vi "Test Functionality.vi"() -> ()   [LabVIEW 2014, in "Exponential Fit Library.lvlib" / "Fit Exponential.lvclass"]
doc: "This is a simle demonstration of the capabilities of the exponential fit class."
uses:
  Fit Exponential.lvclass
  Fit Exponential.lvclass/Fit Exponential.ctl
  Children/DFT1/DFT1.lvclass
  Children/DFT5/DFT5.lvclass
  Children/LRS/LRS.lvclass
  Read Output.vi
  <vilib>/Analysis/1siggen.llb/Ramp Pattern by Delta.vi
  <vilib>/Analysis/NI_AALBase.lvlib
panel:
  out "dt":u32
  out "Fit Output":T1={"e_tau"=99.90454010392875, "tau"=1.949455255190312, "B"=59.81343922735875, "A"=0.8596986263697382}
  in  "B":dbl=2.0
  in  "A":dbl=100.0
  in  "tau":dbl=60.0
  in  "Select Method":enum8{"DFT-1", "DFT-5", "LRS"}(ring)=enum."LRS"
  out "Error in Tau":dbl(graph)=0.8596986263697382
  out "Tau":dbl(graph)=59.81343922735875
  out "Exponential":dbl[](graph)=[105.19602012687483, 88.82122437603577, 94.96086320025637, 95.71453214801636, 95.59080261762062, 91.73977505742936, 85.3376433904598, 82.27233436951714, 84.01552271041503, 77.40281684842637, 81.73542102593571, 85.5916913851243, 79.70119362351942, 73.0659958752437, 78.56339184483366, 78.85934073769867, 67.70414981636233, 76.13121908133753, 69.24243068326123, 75.93686290556164, 63.65334373701221, 78.00875717550242, 70.49870699596495, 75.46168557646813, 72.57838577956375, 65.51622051875438, 65.06989722804512, 65.54430282784585, 55.741189323870316, 54.08478157966374, 54.58255994627164, 64.01000957310953, 50.199772855777525, 65.77049605242452, 54.32498195872571, 62.40495769659772, 60.547552705307, 60.78723411057597, 56.28221634523417, 57.45844769511123, 43.24267064639564, 54.33822050100301, 56.01714381694604, 42.26273032348696, 55.110548218852834, 39.62327233272855, 57.27265986474464, 39.45826734042453, 49.04520882302456, 54.61781894748323, 53.207409848009945, 42.66361091729411, 49.46109003839781, 48.91103509310124, 46.37787029719525, 48.57456698086692, 41.53558769893743, 34.09351700161767, 44.76087587046023, 34.82023460991957, 30.19579831795769, 38.392488493296355, 27.32886941188832, 38.96646638690362, 45.01641242989772, 38.82276973042363, 29.747464621972323, 35.70981436019103, 43.64893196471162, 24.812177457525692, 30.337410961802885, 34.34326852836734, 40.76943704863494, 36.247643405937595, 33.265050395620335, 32.44689219327494, 34.91970637396674, 33.625916966841515, 19.09799738264568, 18.557341036626255, 20.550492201879564, 27.987514461571667, 24.625099541142692, 29.030824648692366, 30.938021456477884, 32.36173983721376, 23.70605502436015, 31.50381194361505, 27.18395847183744, 19.109547699140037, 31.46399815246409, 32.4055920115639, 29.783303066363935, 21.176910913596856, 18.017561362062736, 29.097452111329016, 29.96401325470584, 12.471377487916932, 17.296472399075753, 19.037648942327067, 18.394059462335107, 10.519734089919409, 17.703505869750828, 15.300978961536357, 22.703770314965663, 19.39981126393128, 18.490932701971747, 26.69651222639837, 27.11347151333939, 21.851522164741706, 27.399987380327925, 26.153360943236436, 25.442547503709463, 18.612046341955406, 15.207507655743619, 17.246321867610533, 15.217487467609061, 16.415755701108175, 17.405877185115024, 9.643018876469466, 11.00197276324525, 17.78607754567581, 9.806038474233397, 13.89986279166466, 14.273651492614803, 23.97893894072294, 15.944196378192977, 19.462075911165755, 9.854457059328933, 11.511790216594417, 19.35752907658206, 12.241570925378142, 19.78650740157862, 15.923854316823356, 13.445190057683444, 11.305887529948066, 17.099190329363147, 12.408092598071667, 19.348867839911374, 19.68049621110516, 19.929585723285793, 9.176766049291864, 16.03337774975828, 10.72042467518554, 2.985353813851331, 8.80880342347193, 20.43279328565832, 17.432257850535994, 2.492095373771088, 10.459612835601948, 6.584715449890279, 1.9860289746865192, 8.614572847934767, 13.642779673675129, 7.946713790359805, 8.193726625107967, 3.6747928637811373, 0.1700644620713181, 17.11099515619121, 11.81320739332548, -0.22416290766346236, 1.7775066780920508, 9.00210974722343, 15.442172677636513, 5.795751867202663, 7.291336827842237, 8.46841301371009, 11.568441047889252, 9.08275312271758, 16.747864534855978, 17.384967149474495, -0.2015076152102262, 3.219813909760024, -1.876615029152477, 5.319830410305292, 8.787020848797365, 13.108661073974812, 5.831455321912295, 3.031409258405583, 9.094830744961765, -2.0429697515489886, 12.198360067005474, 13.137788278287854, 7.711897852778436, 8.910334849539328, 13.116022726210625, 8.005563678042822, 5.602355008561599, 4.707261108017689, 15.099479043802113, 13.179981696363699, 15.873888063398443, 14.44212876127556, -2.417352713260132, 3.068148329250591, 4.334067889829247, 13.932329487707698, 12.490687679526246, 8.59216418765527, 4.6017902237449695, -2.1165965418924664, 7.369341116303395, 8.660197758987618, 7.124654530637274, 5.4533104170894315, 8.464662822282104, 1.6463666078431674, 11.055534939521952, 10.99179947366099, 2.955558939130934, 5.308587297714212, 1.5589134301852816, 3.894570060267837, 7.026782289699444, 12.067412422443011, 9.462151640264128, 2.924458692851605, 1.3430994504571796, 10.103720274344525, -3.3027933240387863, 10.830667379215726, 4.656263524636798, 12.063728559375553, -2.8450639772118196, -1.542361677662619, -4.295000715850742, 8.069274106552255, -3.670220056335099, 14.11824716455289, 7.198362554990047, -1.180221561701587, 2.36037908364474, 9.625639667580149, 3.30449161454068, 8.207346401561251, 9.748526464436672, -1.5404232318318627, -1.9282107878049035, 8.974581416440262, 5.555320460489431, 0.9646445190635742, -0.013938779083506603, 9.896315676010175, 3.7290439027482636, 7.91499647577269, 2.0729034768920602, -6.2820431921400655, 13.317043696726468, -3.4617463451476054, 2.968226580706479, -3.385892995971523, 4.971445585809237, -2.3494108824566178, -1.431600043721562, 6.342653303716986, 9.667140392695945, 2.2750657554510285, 6.540922063496764, 13.052883708053669, 2.472313218437308, 8.23422568264313, 13.07017441725549, 1.5895463540372363, 4.037364951378667, -3.073382938680293, 5.6279265661592515, 8.772151967351904, 5.068340037490035, -1.9739269620639277, -1.9545858150530626, 1.80193101241351, 7.556994126436803, 7.257372467882073, -4.177915053957609, 0.7935773029771855, 12.495989410743004, 4.338615925629535, -4.657123763451038, 9.12585580176916, -2.984680608008155, 12.665514777318238, 0.8043741645377445, 7.83894038290061, 3.5075876585542134, -3.646095745298161, 10.86951651939263, 11.79667422876529, 0.7052115458754296, -5.46044302054373, -5.109242070821921, 11.615467865166739, 10.518744795420929, 3.448827352359919, -2.867653489188155, 11.344170344981926, 1.8242103657344118, -6.519381423257056, -3.8721849737221006, -4.394128763132995, 0.18461307524396853, -1.400194685259038, -6.167971018296413, 12.006875538079322, 1.7796915775107869, -6.233014415772429, 7.208797387011845, 4.7749319001285535, 2.8444416782576223, 6.212579213153957, -3.0534074324136724, -1.9026332108746695, -0.567918073437371, -1.9150469645415051, 7.6986289094400995, 3.1390264925905202, 3.4867901827220735, 11.267547229339637, 1.4387042899751372, 11.330200041245975, 6.686456492693113, 0.7436796316430727, 9.520568723046555, -4.764557246173929, -5.9896295659805565, 9.054551460491352, 0.9567665636086242, -6.6850702488225116, 0.050129900114327164, 3.8622815987104215, 8.02710941433822, 2.168693544170771, 0.9615525777552834, 12.27012292943378, 7.75568071336469, -5.288724281618849, 9.725981867123298, -1.9782577492334585, 1.1502239914089705, -2.372657322073878, 3.591898385377584, 11.121780027181533, -4.859527552193626, 8.821766841033481, 8.002308597873029, -5.462720874593407, 8.524752621421822, 8.0238345400469, 2.7582927301824216, 2.3863559871478377, 10.032384812644683, 4.604823589182553, 8.235396713270967, 2.254655955331733, -4.923305371973115, -1.672319360709774, -6.2896697730882885, -6.46553287099009, -2.06281303719418, 10.369248440001929, 11.930578229492795, 8.976202886489983, 11.335966384639635, 9.204318158299069, 11.424734369939998, -4.137947493020789, 0.21215850470936326, 3.1513725327733617, -5.523400415899872, -1.413762810920212, 0.8051270193722377, -1.5496435445287942, -2.0085361877409444, -4.990901398689253, -4.063817234695876, 10.215414274264864, 8.61205246428563, -7.037878789579596, 7.127794087616958, 4.437509493620764, 1.9617703209871546, 6.240843048574737, 3.1158778359359514, 5.267030887712403, -1.6801009281027173, 7.994317867494774, 12.1281099477576, -0.6436646810003808, -0.015314526179357912, 6.727197016398536, -4.863457722675954, -3.6686088288731447, -2.184257590581638, 4.445759286728346, -0.5730726654627412, 11.927046257160521, 7.480923013854309, 6.8767177633984, -1.4351247548297268, -1.9998789173334708, -1.0154114600111757, 7.355599782636551, -3.7495679708350123, 4.891932690590279, -6.391231493286835, -1.1582784155344559, -7.798751488207563, 1.1865985795801164, 11.337219478467388, 5.287748896926077, -7.75671549085444, 1.3609388697503273, -2.9555885013090726, -2.748074107061793, 4.751967496407971, 4.674346934636839, 9.736068739329523, 6.822720712800691, 7.801525091801172, -3.3631144707786995, 7.270211085256085, -5.700906377509993, -2.9938347313397102, 2.512911609426255, -1.605398193902961, -6.192761281670375, 2.8301307990850333, -3.9269839438024663, -6.269066974599594, -4.2169265372943805, -1.2939429717437245, 2.6884567107800486, 2.217048016336004, 6.17411684760568, -3.4911490894388284, 0.013537664399654314, 1.0053912310582207, -0.6433345947522504, 5.520529794416281, -6.94682572871046, 8.801785513704699, -2.974966020074318, 6.672183095054082, -1.5736855353937766, -0.4407090131067828, -4.1775134953567346, -7.885743765943916, 6.0665948776993925, 10.047464667432056, 8.37658076305278, -5.166070638722232, 11.710931802009604, -3.542894873958999, -3.91482479117203, 1.2149385950564096, -6.104643752645355, 6.564532682901516, 9.738835724496106, 10.869155239669801, -3.2786313843496435, -7.853520089121878, -2.0841612526265596, 8.635535692075957, 8.32301228944544, 2.4872620812023656, -2.630515978073298, 4.232129898169866, -0.6516605674184142, 11.468863752506813, 7.7853362781960005, -5.273961006323416, -7.84466275996577, 4.447067560217456, 1.4988354295623267, 1.2822836361101038, 4.06504393901003, 2.853860535955336, 6.586118316530074, -7.12265315261501, -4.688320282040835, -4.16899208896246, -3.477799101705977, -6.503236651736497, 0.9649265143561232, 6.965570382111784, -5.902112018352068, -5.461486656362075, 10.704711602129656, -6.198637863129425, 2.5263212458413693, -2.491843920438005, -6.3695628659412105, -2.9250324471878955, 4.093421529221677, 0.13373864125033208, -5.744432219975616, 11.567219626840865, -1.4608501743895266, 10.736569515034251, 10.141100006738567, -0.4997728969080599]
  # "Exponential Input"
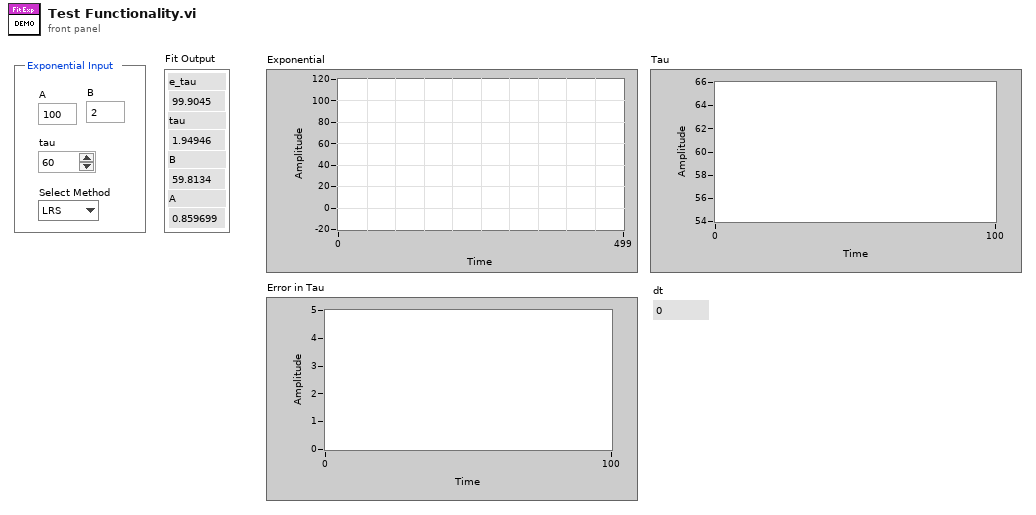
[diagram p1: front panel]
types:
  T1 = cluster{"e_tau":dbl, "tau":dbl, "B":dbl, "A":dbl}
  T2 = cluster{"A":dbl, "B":dbl, "tau":dbl, "e_tau":dbl}
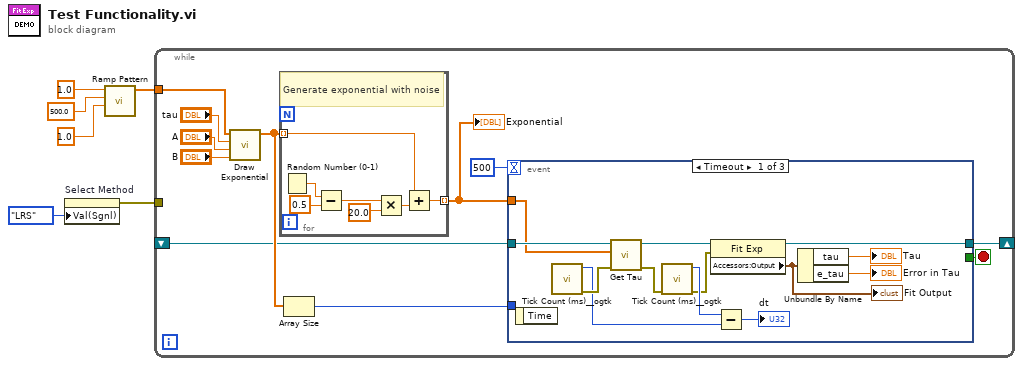
[diagram p0: block diagram]
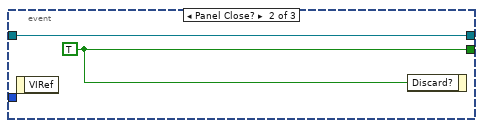
[diagram p2: hidden frame]
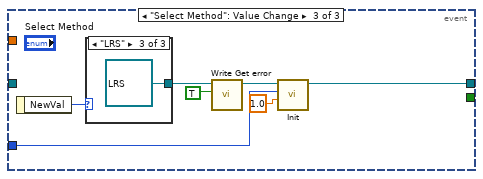
[diagram p3: hidden frame]
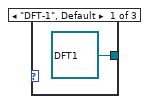
[diagram p4: hidden frame]
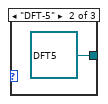
[diagram p5: hidden frame]
diagram:
  n1 = property on="Select Method" class="Enum (strict)"("Val(Sgnl)"=enum8{"DFT-1", "DFT-5", "LRS"}."LRS" ("Value (Signaling)")) -> (error out=w1:errorcluster)  [unwired: 2 in, 1 out]
  n2 = call-poly <vilib>:"Ramp Pattern.vi"("start"=1.0, "end"=500.0, "delta"=1.0) -> ("Ramp Pattern"=w3:dbl[])  [unwired: 6 in, 2 out]
  n3 = while {
    tunnel: w3 -> [w17]
    shift-right: [w13] -> _
    shift-left: _ -> [w9]
    tunnel: w1 -> [_]
    stop <- w7 stop-if-true
    n4 = call "Draw Exponential.vi"("B"="B", "A"="A", "tau"="tau", "time"=w17) -> ("ExponentialOut"=w12:dbl[])  [unwired: 7 in]
    n5 = for {
      tunnel: w12 -> [w44] mode=indexing
      tunnel: [w43] -> w8 mode=indexing
      # "Generate exponential with noise"
      n6 = Random Number (0-1)() -> (number: 0 to 1=w49:dbl)
      n7 = Subtract(x=w49, y=0.5) -> (x-y=w47:dbl)
      n8 = Multiply(x=w47, y=20.0) -> (x*y=w45:dbl)
      n9 = Add(x=w44, y=w45) -> (x+y=w43:dbl)
    }
    "Exponential" <- w8
    n10 = Array Size(array=w12) -> (size(s)=w11:i32)
    n11 = event shown="[0] Timeout" {
      selector: _ -> [_ _ _]
      dyn-events: _ -> [_ _ _]
      timeout: 500 -> [_ _ _]
      tunnel: [w28 w31 w38] -> w13
      tunnel: w11 -> [_ _ w37]
      tunnel: w9 -> [w30 w31 _]
      tunnel: w8 -> [w27 _ _]
      tunnel: [_ w32 _] -> w7
      event Timeout {
        n12 = event-data() -> ()  [unwired: 1 in, 1 out]
        n13 = call <userlib>:"Tick Count (ms)__ogtk.vi"() -> ("error out"=w22:errorcluster, "millisecond timer value"=w20:u32)  [unwired: 10 in]
        n14 = call "Get Tau.vi"("error in"=w22, "Data In"=w27, "Fit Exp in"=w30) -> ("error out"=w23:errorcluster, "Fit Exp out"=w29:refnum<class "Fit Exponential.lvclass">)  [unwired: 7 in]
        n15 = call <userlib>:"Tick Count (ms)__ogtk.vi"("error in (no error)"=w23) -> ("error out"=w18:errorcluster, "millisecond timer value"=w21:u32)  [unwired: 9 in]
        n16 = property class="Fit Exp"(reference=w29, error in=w18) -> (reference out=w28:refnum<class "Fit Exponential.lvclass">, "Accessors:Output"=w24:T2)  [unwired: 1 out]
        "Fit Output" <- w24
        n17 = Subtract(x=w21, y=w20) -> (x-y=→"dt":u32)
        n18 = Unbundle By Name(w24) -> ("tau"=→"Tau":dbl, "e_tau"=→"Error in Tau":dbl)
      }
      event Panel Close? {
        w32 = TRUE
        n19 = event-data() -> ()  [unwired: 1 in, 1 out]
        n20 = event-data("Discard?"=w32) -> ()  [unwired: 1 in, 1 out]
      }
      event "Select Method": Value Change {
        n21 = event-data() -> ("NewVal"=w39:enum8{"DFT-1", "DFT-5", "LRS"})  [unwired: 1 in]
        n22 = case shown="\"LRS\"" w39 {
          tunnel: [refnum<class "DFT1.lvclass"> refnum ("Exponential Fit Library.lvlib:DFT-1") refnum<class "DFT5.lvclass"> refnum ("Exponential Fit Library.lvlib:DFT-5") refnum<class "LRS.lvclass"> refnum ("Exponential Fit Library.lvlib:LRS")] -> w35
          frame "DFT-1", Default {
          }
          frame "DFT-5" {
          }
          frame "LRS" {
          }
        }
        n23 = call "Write Get error.vi"("Get error?"=TRUE, "Fit Exponential in"=w35) -> ("Fit Exponential out"=w34:refnum<class "Fit Exponential.lvclass">)  [unwired: 8 in, 1 out]
        n24 = call-dynamic "Init.vi"("Dt"=1.0, "Size"=w37, "Fit Exponential in"=w34) -> ("Fit Exponential out"=w38:refnum<class "Fit Exponential.lvclass">)  [unwired: 8 in]
      }
    }
  }
